vi "Demo EV3-OnShape.vi"() -> ()   [LabVIEW 2019]
uses:
  _SubVI/default document.vi
  <userlib>/Onshape Feature Functions/_SubVI/FS Body Cuboid.vi
panel:
  in  "Cuboid":T1={"Point 1"={"x"=0.0, "y"=0.0, "z"=0.0}, "Point 2"={"x"=1.0, "y"=1.0, "z"=1.0}}
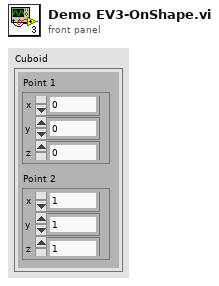
[diagram p1: front panel]
types:
  T1 = cluster{"Point 1":cluster{"x":dbl, "y":dbl, "z":dbl}, "Point 2":cluster{"x":dbl, "y":dbl, "z":dbl}}
  T2 = cluster{"y1":i32, "x1":i32, "x2":i32, "y2":i32, "extrude":i32, "setflag":string}
  T3 = typedef "Cluster.ctl" = cluster{"Date":string, "On-Nonce":string, "eid":string, "wid":string, "did":string, "name":string, "method":string, "Accept":string, "User-Agent":string, "Content-Type":string, "stack":string, "headers":string[], "payload":string, "ctype":string, "path":string, "Authorization":string, "secret_key":string, "access_key":string}
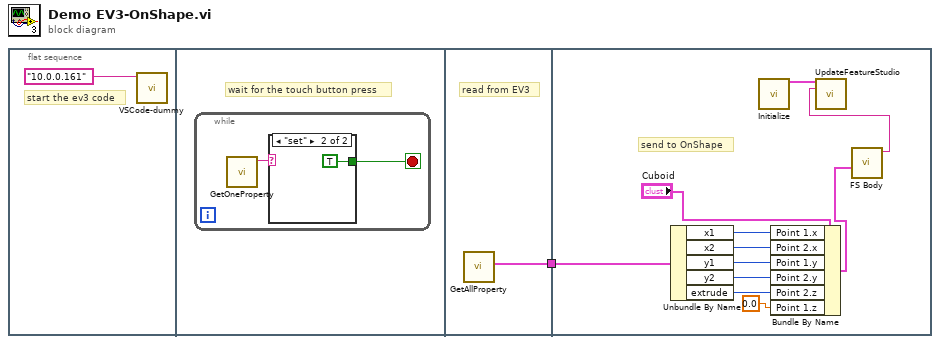
[diagram p0: block diagram]
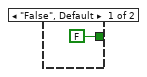
[diagram p2: hidden frame]
diagram:
  n1 = flat-sequence {
    tunnel: [w7] -> w1
    tunnel: w1 -> [w17]
    frame #0 {
      # "start the ev3 code"
      n2 = call "VSCode-dummy.vi"("Enter your IP address"="10.0.0.161") -> ()  [unwired: 9 in, 2 out]
    }
    frame #1 {
      # "wait for the touch button press"
      n3 = while {
        stop <- w3 stop-if-true
        n4 = call "GetOneProperty.vi"() -> ("setflag"=w4:string)  [unwired: 10 in, 1 out]
        n5 = case shown="\"set\"" w4 {
          tunnel: [FALSE TRUE] -> w3
          frame "False", Default {
          }
          frame "set" {
          }
        }
      }
    }
    frame #2 {
      # "read from EV3"
      n6 = call "GetAllProperty.vi"() -> ("element"=w7:T2)  [unwired: 10 in, 1 out]
    }
    frame #3 {
      # "send to OnShape"
      n7 = Unbundle By Name(w17) -> ("x1"=w15:i32, "x2"=w14:i32, "y1"=w13:i32, "y2"=w12:i32, "extrude"=w11:i32)
      n8 = call-poly "Initialize.vi"() -> ("Device Out"=w18:T3)  [unwired: 13 in, 2 out]
      n9 = Bundle By Name(cluster="Cuboid", "Point 1.x"=w15, "Point 2.x"=w14, "Point 1.y"=w13, "Point 2.y"=w12, "Point 2.z"=w11, "Point 1.z"=0.0) -> (w9:T1)
      n10 = call-poly <userlib>:"FS Body.vi"("Cuboid"=w9) -> ("Feature Out"=w8:string)  [unwired: 10 in]
      n11 = call <userlib>:"UpdateFeatureStudio.vi"("Device In"=w18, "FeatureScript"=w8) -> ()  [unwired: 11 in, 3 out]
    }
  }
